vi "Read Channel scanner configuration.vi"(8 "error in (no error)":errorcluster, 11 "Channel Scanner in":refnum<class "Channel Scanner.lvclass">) -> (0 "error out":errorcluster, 2 "Configuration":T1, 3 "Channel Scanner out":refnum<class "Channel Scanner.lvclass">)   [LabVIEW 2016, in "Channel Scanner.lvclass"]
uses:
  Channel Scanner.lvclass
  C:/github/LabActor/Template Module/Template Module.lvclass
  Channel Scanner Configuration.ctl
  Template Module/Template Module.lvclass/Template Module.ctl
  Template Module/Read Configuration.vi
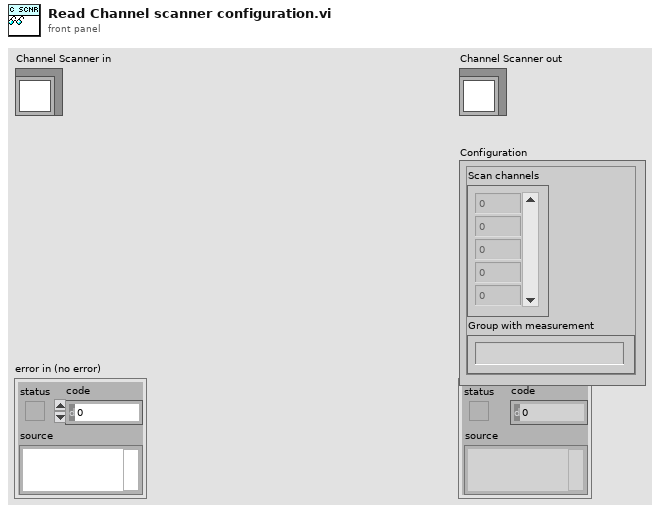
[diagram p1: front panel]
types:
  T1 = typedef "Channel Scanner Configuration.ctl" = cluster{"Scan channels":i32[], "Group with measurement":string}
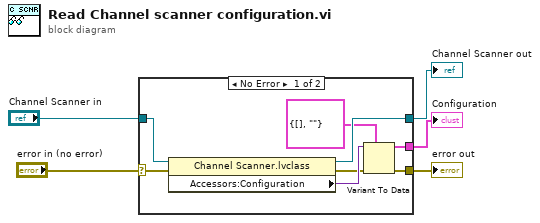
[diagram p0: block diagram]
diagram:
  n1 = case shown="No Error" "error in (no error)" {
    selector: "error in (no error)" -> [w7 w14]
    tunnel: [w11 w14] -> w4
    tunnel: [w12 w15] -> w2
    tunnel: "Channel Scanner in" -> [w13 w15]
    tunnel: [w6 _] -> w1
    frame No Error {
      n2 = property class="Channel Scanner.lvclass"(reference=w13, error in=w7) -> (reference out=w12:refnum<class "Channel Scanner.lvclass">, error out=w8:errorcluster, "Accessors:Configuration"=w9:variant)
      n3 = Variant To Data(error in=w8, type=T1 {"Scan channels"=[], "Group with measurement"=""} ("Channel scanner configuration"), Variant=w9) -> (data=w6:T1, error out=w11:errorcluster)
    }
    frame Error {
    }
  }
  "error out" <- w4
  "Channel Scanner out" <- w2
  "Configuration" <- w1
